vi "OutputCompressor.vi"   [LabVIEW 2020]
doc: "This VI sends commands to the compressor."
uses:
  refnums.vi
  GRNF_Compressor.vi
  dsdata.vi
types:
  T1 = typedef "WPI_CompressorDevRef.ctl" = cluster{"DevStatus":errorcluster, "Pneumatics Control Module":u8}
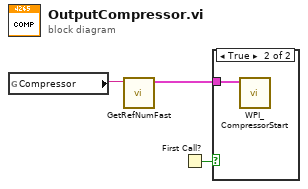
[diagram p0: block diagram]
diagram:
  n1 = global read "refnums.vi" "Compressor"() -> (w2:string)
  n2 = call-poly "GetRefNumFast.vi"("RefNum Name"=w2) -> ("Device Reference"=w3:T1)  [unwired: 5 in, 1 out]
  n3 = First Call?() -> (First Call?: T/F=w1:bool)
  n4 = case shown="True" w1 {
    tunnel: w3 -> [_ w4]
    frame False {
    }
    frame True {
      n5 = call <vilib>:"WPI_CompressorStart.vi"("CompressorDevRef"=w4) -> ()  [unwired: 9 in, 2 out]
    }
  }
